vi "Test Vectors (SHA-1).vi"() -> (3 "All Vectors passed":bool)   [LabVIEW 2013]
uses:
  src/SHA-1 Pad.vi
  src/SHA-1 Core.vi
  src/SHA-1 Digest.vi
  src/SHA-1.lvlib
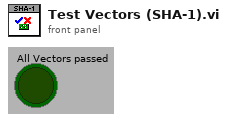
[diagram p1: front panel]
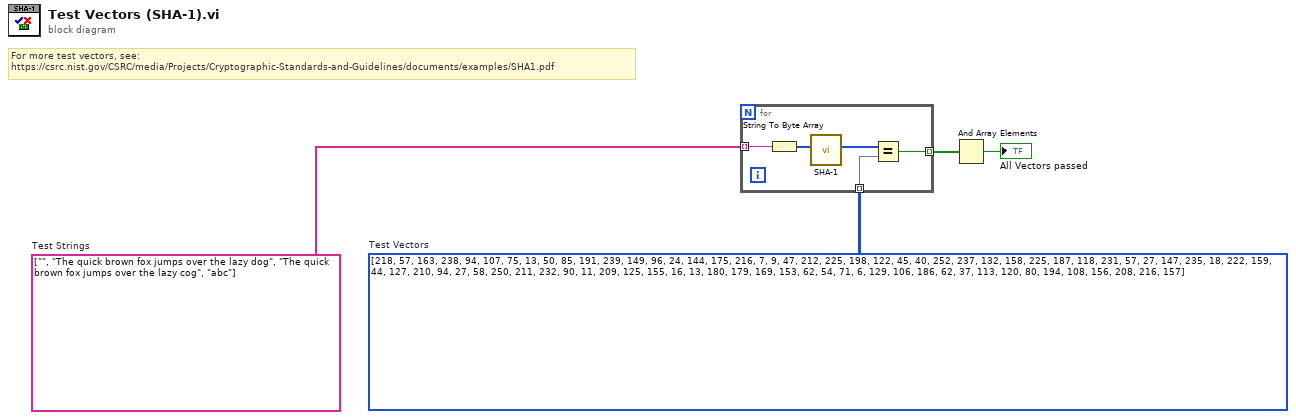
[diagram p0: block diagram]
diagram:
  w4 = string[] ["", "The quick brown fox jumps over the lazy dog", "The quick brown fox jumps over the lazy cog", "abc"]  # Test Strings
  w3 = u8[][] [[218, 57, 163, 238, 94, 107, 75, 13, 50, 85, 191, 239, 149, 96, 24, 144, 175, 216, 7, 9], [47, 212, 225, 198, 122, 45, 40, 252, 237, 132, 158, 225, 187, 118, 231, 57, 27, 147, 235, 18], [222, 159, 44, 127, 210, 94, 27, 58, 250, 211, 232, 90, 11, 209, 125, 155, 16, 13, 180, 179], [169, 153, 62, 54, 71, 6, 129, 106, 186, 62, 37, 113, 120, 80, 194, 108, 156, 208, 216, 157]]  # Test Vectors
  # "For more test vectors, see:\nhttps://csrc.nist.gov/CSRC/media/Projects/Cryptographic-Standards-and-Guidelines/documents/examples/SHA1.pdf"
  n1 = for {
    tunnel: w4 -> [w9] mode=indexing
    tunnel: w3 -> [w8] mode=indexing
    tunnel: [w7] -> w2 mode=indexing
    n2 = String To Byte Array(string=w9) -> (unsigned byte array=w6:u8[])
    n3 = call "SHA-1.vi"("Data"=w6) -> ("message-digest"=w5:u8[])  [unwired: 10 in]
    n4 = Equal?(x=w5, y=w8) -> (x = y?=w7:bool)
  }
  n5 = And Array Elements(Boolean array=w2) -> (logical AND=→"All Vectors passed":bool)
